vi "TDMS_Logging_Loop.vi"(6 "Logging Period (ms)":i64=20, 7 "Buffer Size":u32=1000, 9 "Group Initialization":T2(array[cluster]), 10 "TDMS Name":string="Test", 11 "Log to USB?":bool) -> ()   [LabVIEW 2015]
uses:
  <userlib>/836-Library/System/TDMSv2/Group_Data.ctl
  <userlib>/836-Library/System/TDMSv2/Group_Channels.ctl
  <userlib>/836-Library/System/TDMSv2/TDMS_RT_FIFO_Packet.ctl
  <userlib>/836-Library/System/TDMSv2/Channel_Initializer.ctl
  <vilib>/Platform/TimedLoop/XDataNode/timing_clust.ctl
  <vilib>/Platform/TimedLoop/XDataNode/nitl_modes.ctl
  <vilib>/Platform/TimedLoop/XDataNode/wakeup.ctl
  <userlib>/836-Library/System/TDMSv2/Back_Channel_Data.ctl
  <vilib>/platform/TimedLoop/XDataNode/XDataNode.xnode
  <vilib>/Platform/TimedLoop/XDataNode/XDNodeRunTimeDep.lvlib
panel:
  out "Logging Iteration Count":i32
  out "TDMS Name":string="Test"
  out "File Creation Loop Iteration":i32
  out "Current Data":T1
  out "TDMS File Location":path
  out "Cluster 2":T5
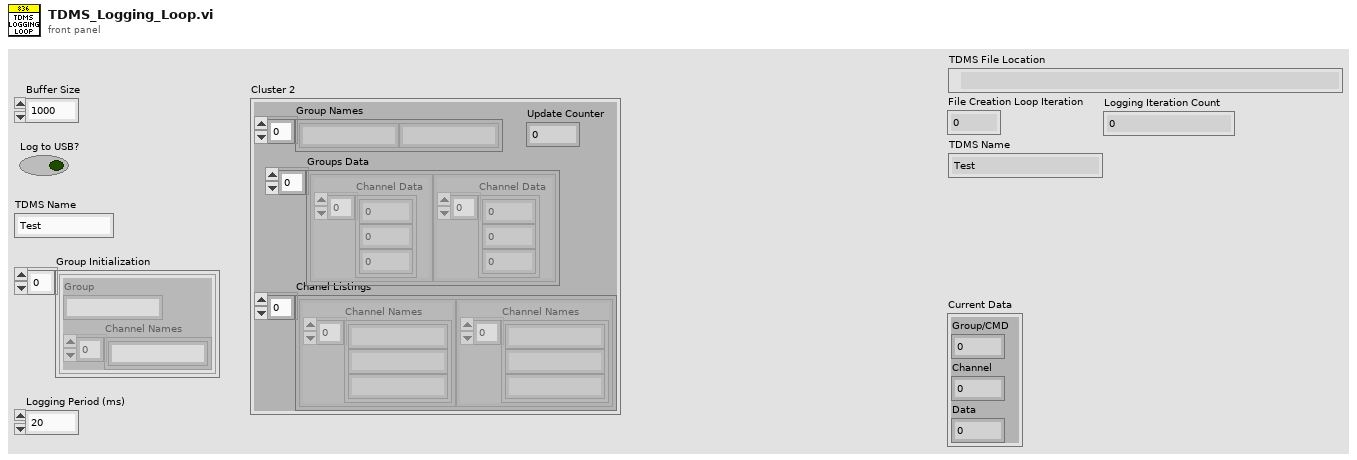
[diagram p1: front panel]
types:
  T1 = typedef "TDMS_RT_FIFO_Packet.ctl" = cluster{"Group/CMD":i32, "Channel":i32, "Data":dbl}
  T2 = cluster{"Group":string, "Channel Names":string[]}[]
  T3 = typedef "Group_Data.ctl" = cluster{"Channel Data":dbl[]}
  T4 = typedef "Group_Channels.ctl" = cluster{"Channel Names":string[]}
  T5 = cluster{"Group Names":string[], "Groups Data":T3[], "Update Counter":i32, "Chanel Listings":T4[]}
  T6 = enum16{"open", "open or create", "create or replace", "create", "open (read-only)"}
  T7 = typedef "XDNodeRunTimeDep.lvlib/timing_clust.ctl" = cluster{"Expected End [f-1]":u64, "Actual End [f-1]":u64, "Finished Late? [f-1]":bool, "Expected End [i-1]":u64, "Actual End [i-1]":u64, "Finished Late? [i-1]":bool, "Expected Start [i]":u64, "Actual Start [i]":u64, "Expected Start [f]":u64, "Actual Start [f]":u64, "Source Name":string, "Structure Name":string, "Period":i64, "Deadline":i64, "Offset":i64, "Start":i64, "Priority":i32, "Timeout":i32, "Mode":T8, "Wakeup Reason":T9, "Error":errorcluster, "Source Type":string, "Secondary Source Type":string, "Global End Time":u64, "Global Start Time":u64, "Frame Duration":u64, "Iteration Duration":u64, "Assigned CPU":i32, "I/O Scan Engine Mode":u32}
  T8 = typedef "XDNodeRunTimeDep.lvlib/nitl_modes.ctl" = enum32{"No Change", "Process missed periods, maintain original phase", "Discard missed periods, maintain original phase", "Process missed periods, ignore original phase", "Discard missed periods, ignore original phase"}
  T9 = typedef "XDNodeRunTimeDep.lvlib/wakeup.ctl" = enum32{"Normal", "Aborted", "Asynchronous wakeup", "Timing source error", "Timed loop error", "Timeout"}
  T10 = typedef "Channel_Initializer.ctl" = cluster{"Column Headers":string[], "Initialization array":dbl[]}
  T11 = typedef "Back_Channel_Data.ctl" = cluster{"Group":string, "Channel":string, "Return Notifier":refnum<notifier>}
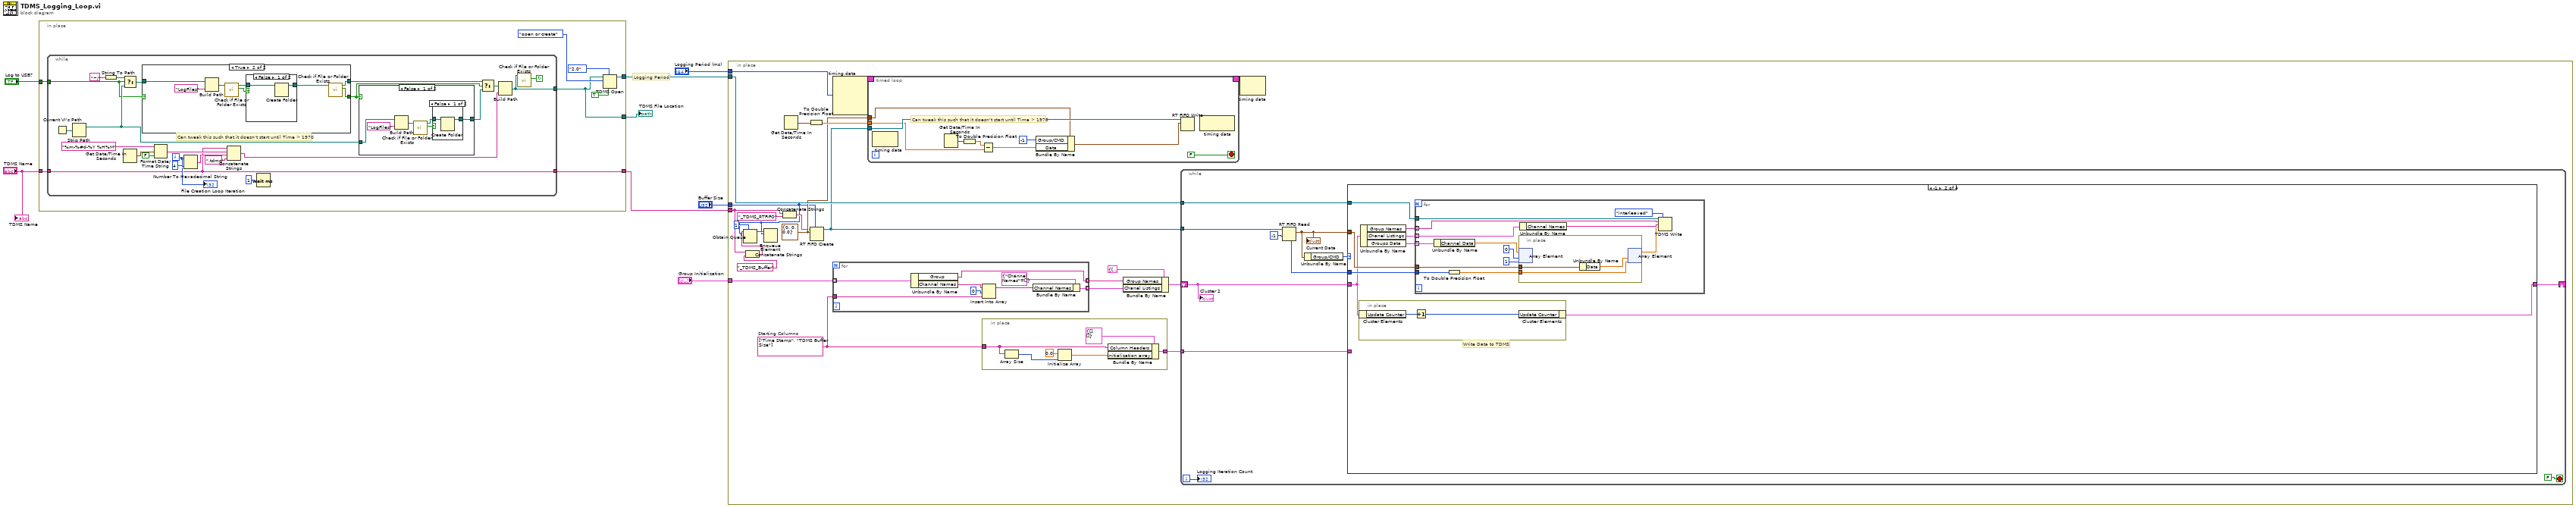
[diagram p0: block diagram]
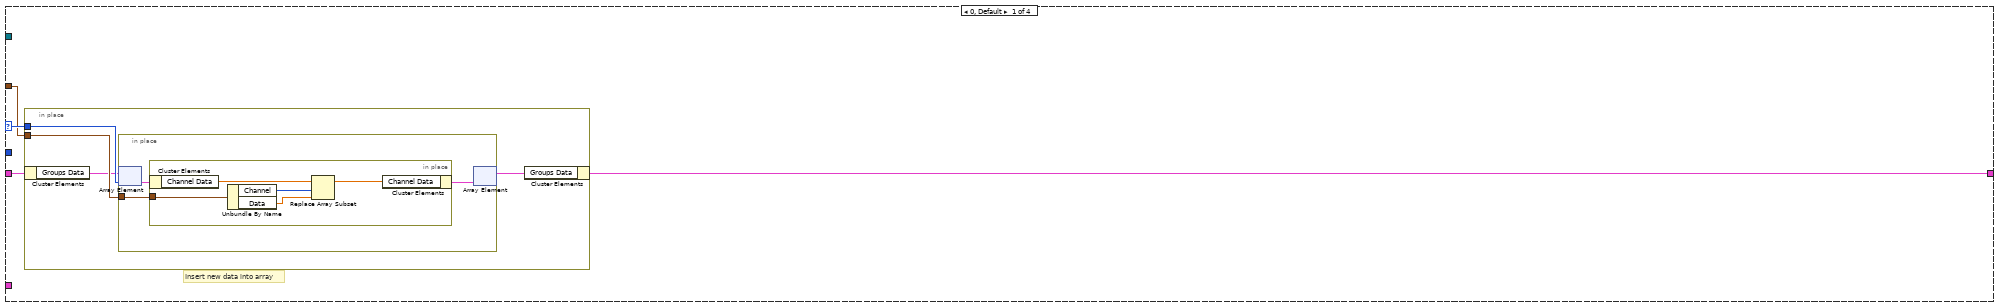
[diagram p6: hidden frame]
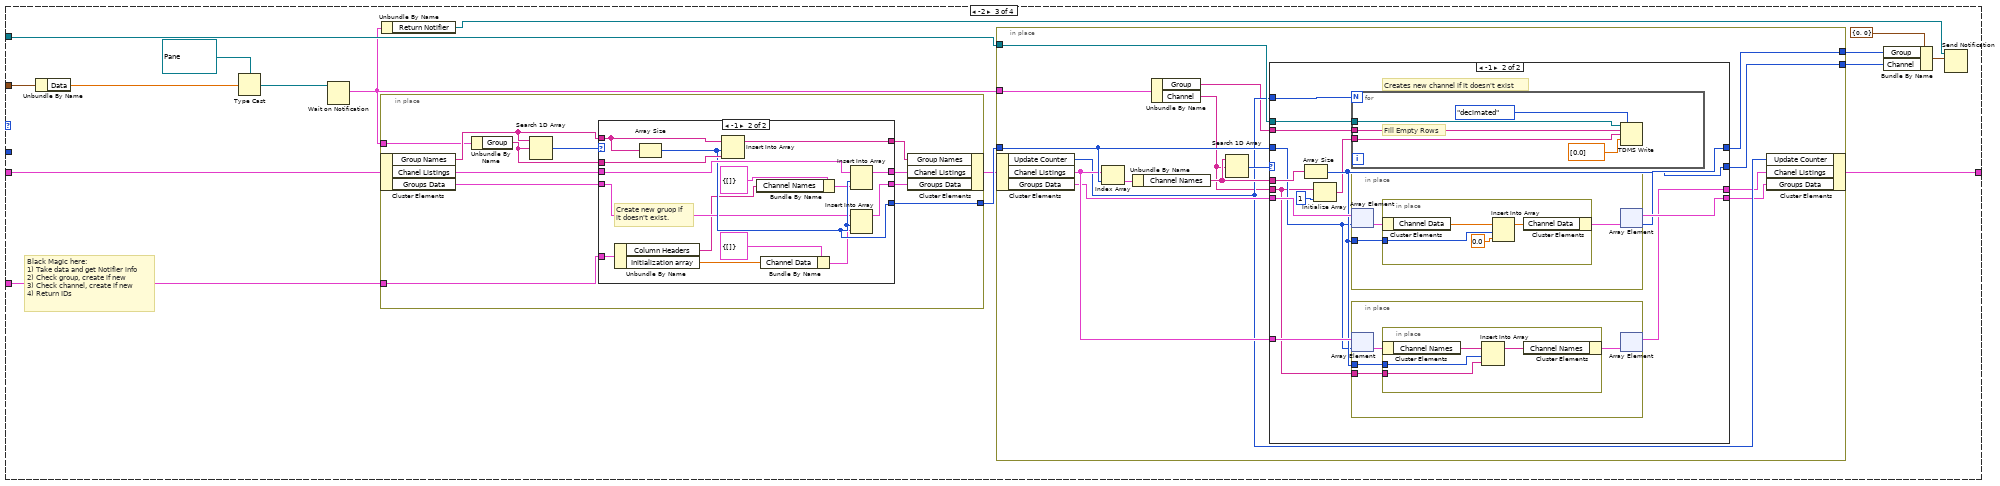
[diagram p7: hidden frame]
diagram:
  # "Logging Period"
  n1 = in-place {
    in-place-border: [w11] -> w2
    in-place-border: "Log to USB?" -> [w13]
    in-place-border: "TDMS Name" -> [w12]
    in-place-border: [w10] -> w5
    in-place-border: [w9] -> w1
    n2 = while {
      tunnel: [w29] -> w9
      tunnel: w13 -> [w18]
      tunnel: w12 -> [w17]
      tunnel: [w17] -> w10
      i -> [w33]
      stop <- w30 continue-if-true
      # "Can tweak this such that it doesn't start until Time > 1970"
      n3 = Current VI's Path() -> (path=w28:path)
      n4 = Strip Path(path=w28) -> (stripped path=w22:path)  [unwired: 1 out]
      n5 = String To Path(string="~/") -> (path=w26:path)
      n6 = Select(t=w26, s=w18, f=w22) -> (s? t:f=w27:path)
      n7 = Get Date/Time In Seconds() -> (seconds since 1Jan1904=w35:timestamp)
      n8 = case shown="True" w18 {
        selector: w18 -> [w41 _]
        tunnel: w27 -> [w40 w46]
        tunnel: [w40 w43] -> w24
        tunnel: [w41 w42] -> w21
        frame False {
        }
        frame True {
          n9 = Build Path(base path=w46, name or relative path="LogFiles") -> (appended path=w45:path)
          n10 = call <vilib>:"Check if File or Folder Exists.vi"("path"=w45) -> ("file or folder exists?"=w49:bool, "dup path"=w48:path)  [unwired: 8 in, 1 out]
          n11 = case shown="False" w49 {
            tunnel: [w51 w52] -> w44
            tunnel: w48 -> [w50 w52]
            frame False {
              n12 = Create Folder(path (use dialog)=w50) -> (created path=w51:path)  [unwired: 2 in, 2 out]
            }
            frame True {
            }
          }
          n13 = call <vilib>:"Check if File or Folder Exists.vi"("path"=w44) -> ("file or folder exists?"=w42:bool, "dup path"=w43:path)  [unwired: 8 in, 1 out]
        }
      }
      n14 = Format Date/Time String(time format string (%c)="%m-%#d-%Y %H%M", seconds (now)=w35, UTC format=FALSE) -> (date/time string=w38:string)
      n15 = Number To Hexadecimal String(1:i16 4 ("width (-)"), 2:w33) -> (0:w31:string)
      n16 = Concatenate Strings(w17, w38, w31, ".tdms" ("string")) -> (w39:string)
      n17 = Wait (ms)(milliseconds to wait=u32 1 ("millisecond multiple")) -> ()  [unwired: 1 out]
      n18 = case shown="False" w21 {
        tunnel: w22 -> [w57 w62]
        tunnel: [w53 w62] -> w20
        frame False {
          n19 = Build Path(base path=w57, name or relative path="LogFiles") -> (appended path=w54:path)
          n20 = call <vilib>:"Check if File or Folder Exists.vi"("path"=w54) -> ("file or folder exists?"=w55:bool, "dup path"=w56:path)  [unwired: 8 in, 1 out]
          n21 = case shown="False" w55 {
            tunnel: [w60 w61] -> w53
            tunnel: w56 -> [w59 w61]
            frame False {
              n22 = Create Folder(path (use dialog)=w59) -> (created path=w60:path)  [unwired: 2 in, 2 out]
            }
            frame True {
            }
          }
        }
        frame True {
        }
      }
      n23 = Select(t=w24, s=w21, f=w20) -> (s? t:f=w23:path)
      n24 = Build Path(base path=w23, name or relative path=w39) -> (appended path=w29:path)
      n25 = call <vilib>:"Check if File or Folder Exists.vi"("path"=w29) -> ("file or folder exists?"=w30:bool)  [unwired: 8 in, 2 out]
      "File Creation Loop Iteration" <- w33
    }
    n26 = TDMS Open(6:TRUE ("disable buffering? (T)"), 7:enum16{"1.0", "2.0"}."2.0" ("file format version (2.0)"), 10:T6."open or create" ("operation (0:open)"), 11:w9) -> (3:w11:refnum<k34>)  [unwired: 3 in, 1 out]
  }
  "TDMS File Location" <- w1
  n27 = in-place {
    in-place-border: w2 -> [w85]
    in-place-border: "Logging Period (ms)" -> [w81]
    in-place-border: w5 -> [w68]
    in-place-border: "Buffer Size" -> [w63]
    in-place-border: "Group Initialization" -> [w78]
    w73 = string[] ["Time Stamp", "TDMS Buffer Size"]  # Starting Columns
    w80 = T1 {"Group/CMD"=0, "Channel"=0, "Data"=0.0}
    n28 = Concatenate Strings(w68, "_TDMS_Buffer" ("string")) -> (w67:string)
    n29 = Obtain Queue(max queue size (-1, unlimited)=1, name (unnamed)=w67, element data type=w63) -> (queue out=w64:refnum<queue>)  [unwired: 2 in, 2 out]
    n30 = Enqueue Element(queue=w64, element=w63) -> ()  [unwired: 2 in, 3 out]
    n31 = Concatenate Strings(w68, "_TDMS_RTFIFO" ("string")) -> (w72:string)
    n32 = Get Date/Time In Seconds() -> (seconds since 1Jan1904=w82:timestamp)
    n33 = To Double Precision Float(number=w82) -> (double precision float=w83:dbl)
    n34 = RT FIFO Create(0:w72, 1:w80, 4:w63) -> (8:w84:refnum<k33>)  [unwired: 5 in, 2 out]
    n35 = node-c288(w81) -> (w70:T7)  [unwired: 3 in]
    n36 = for {
      tunnel: w78 -> [w108] mode=indexing
      tunnel: [w107] -> w76 mode=indexing
      tunnel: [w104] -> w74 mode=indexing
      tunnel: w73 -> [w101]
      n37 = Unbundle By Name(w108) -> ("Group"=w107:string, "Channel Names"=w106:string[])
      n38 = Insert Into Array(array=w106, index=0, new element=w101) -> (w103:string[])
      n39 = Bundle By Name(cluster=T4 {"Channel Names"=[]}, "Channel Names"=w103) -> (w104:T4)
    }
    n40 = timed-loop {
      timing: w70 -> [_]
      timing-out: [_] -> w69
      tunnel: w84 -> [w93]
      tunnel: w80 -> [w92]
      tunnel: w83 -> [w86]
      stop <- FALSE stop-if-true
      # "Can tweak this such that it doesn't start until Time > 1970"
      n41 = node-c288() -> ()  [unwired: 1 in, 1 out]
      n42 = Get Date/Time In Seconds() -> (seconds since 1Jan1904=w89:timestamp)
      n43 = To Double Precision Float(number=w89) -> (double precision float=w88:dbl)
      n44 = Subtract(x=w88, y=w86) -> (x-y=w87:dbl)
      n45 = Bundle By Name(cluster=w92, "Group/CMD"=-1 ("Index/CMD"), "Data"=w87) -> (w91:T1)
      n46 = RT FIFO Write(0:w93, 1:w91) -> ()  [unwired: 3 in, 4 out]
      n47 = node-c288() -> ()  [unwired: 1 in, 1 out]
    }
    n48 = in-place {
      in-place-border: w73 -> [w110]
      in-place-border: [w109] -> w79
      n49 = Array Size(array=w110) -> (size(s)=w113:i32)
      n50 = Initialize Array(0.0 ("element"), w113) -> (w111:dbl[])
      n51 = Bundle By Name(cluster=T10 {"Column Headers"=[], "Initialization array"=[]} ("Column Initializer"), "Column Headers"=w110, "Initialization array"=w111) -> (w109:T10)
    }
    n52 = Bundle By Name(cluster=T5 {"Group Names"=[], "Groups Data"=[], "Update Counter"=0, "Chanel Listings"=[]}, "Group Names"=w76, "Chanel Listings"=w74) -> (w75:T5)
    n53 = while {
      tunnel: w85 -> [w125]
      tunnel: w84 -> [w123]
      tunnel: w79 -> [w119]
      shift-right: [w116] -> _
      shift-left: w75 -> [w117]
      i -> [w115]
      stop <- FALSE stop-if-true
      n54 = RT FIFO Read(0:w123, 2:-1 ("timeout in ms (0)")) -> (7:w121:u32, 9:w118:T1)  [unwired: 2 in, 3 out]
      "Current Data" <- w118
      n55 = Unbundle By Name(w118) -> ("Group/CMD"=w122:i32)
      n56 = case shown="-1" w122 {
        selector: w122 -> [w129 _ _ _]
        tunnel: w125 -> [_ w149 w176 _]
        tunnel: w121 -> [_ w148 _ _]
        tunnel: w119 -> [_ _ w175 _]
        tunnel: w118 -> [w128 w147 w174 _]
        tunnel: w117 -> [w127 w143 w172 w267]
        tunnel: [w126 w142 w170 w267] -> w116
        frame 0, Default {
          # "Insert new data into array"
          n57 = in-place {
            in-place-border: w129 -> [w133]
            in-place-border: w128 -> [w132]
            n58 = in-place-cluster #1(w127) -> ("Groups Data"=w131:T3[])
            n59 = in-place {
              in-place-border: w132 -> [w134]
              n60 = in-place-array #2(w131, w133) -> (w136:T3)
              n61 = in-place {
                in-place-border: w134 -> [w139]
                n62 = in-place-cluster #3(w136) -> ("Channel Data"=w141:dbl[])
                n63 = Unbundle By Name(w139) -> ("Channel"=w138:i32, "Data"=w137:dbl)
                n64 = Replace Array Subset(array=w141, new element=w137, index=w138) -> (w140:dbl[])
                n65 = in-place-cluster #3("Channel Data"=w140) -> (w135:T3)
              }
              n66 = in-place-array #2(w135) -> (w130:T3[])  [unwired: 1 out]
            }
            n67 = in-place-cluster #1("Groups Data"=w130) -> (w126:T5)
          }
        }
        frame -1 {
          # "Write Data to TDMS"
          n68 = in-place {
            n69 = in-place-cluster #4(w143) -> ("Update Counter"=w151:i32)
            n70 = Increment(x=w151) -> (x+1=w150:i32)
            n71 = in-place-cluster #4("Update Counter"=w150) -> (w142:T5)
          }
          n72 = Unbundle By Name(w143) -> ("Group Names"=w144:string[], "Chanel Listings"=w146:T4[], "Groups Data"=w145:T3[])
          n73 = for {
            tunnel: w149 -> [w164]
            tunnel: w145 -> [w163] mode=indexing
            tunnel: w146 -> [w162] mode=indexing
            tunnel: w144 -> [w161] mode=indexing
            tunnel: w148 -> [w160]
            tunnel: w147 -> [w152]
            n74 = Unbundle By Name(w163) -> ("Channel Data"=w157:dbl[])
            n75 = To Double Precision Float(number=w160) -> (double precision float=w154:dbl)
            n76 = in-place {
              in-place-border: w154 -> [w167]
              in-place-border: w152 -> [w166]
              n77 = in-place-array #5(w157, 0, 1) -> ()  [unwired: 2 out]
              n78 = Unbundle By Name(w166) -> ("Data"=w165:dbl)
              n79 = in-place-array #5(w165, w167) -> (w153:dbl[])  [unwired: 2 out]
            }
            n80 = Unbundle By Name(w162) -> ("Channel Names"=w159:string[])
            n81 = TDMS Write(0:w164, 1:enum16{"decimated", "interleaved"}."interleaved" ("data layout (0:decimated)"), 5:w161, 7:w159, 9:w153) -> ()  [unwired: 1 in, 4 out]
          }
        }
        frame -2 {
          # "Black Magic here:\n1) Take data and get Notifier info\n2) Check group, create if new\n3) Check channel, create if new\n4) Return IDs"
          n82 = Unbundle By Name(w174) -> ("Data"=w173:dbl)
          n83 = Type Cast(type=refnum<notifier> refnum ("notifier out"), x=w173) -> (*(type *) &x=w182:refnum<notifier>)
          n84 = Wait on Notification(notifier=w182) -> (notification=w168:T11)  [unwired: 3 in, 3 out]
          n85 = in-place {
            in-place-border: [w246] -> w178
            in-place-border: w175 -> [w245]
            in-place-border: w168 -> [w238]
            n86 = in-place-cluster #6(w172) -> ("Group Names"=w244:string[], "Chanel Listings"=w240:T4[], "Groups Data"=w242:T3[])
            n87 = Unbundle By Name(w238) -> ("Group"=w237:string)
            n88 = Search 1D Array(1D array=w244, element=w237) -> (index of element=w247:i32)  [unwired: 1 in]
            n89 = case shown="-1" w247 {
              selector: w247 -> [w251 _]
              tunnel: w244 -> [w250 w266]
              tunnel: w237 -> [_ w265]
              tunnel: [w251 w262] -> w246
              tunnel: [w250 w264] -> w243
              tunnel: w240 -> [w249 w263]
              tunnel: w242 -> [w248 w261]
              tunnel: [w249 w260] -> w239
              tunnel: [w248 w259] -> w241
              tunnel: w245 -> [_ w254]
              frame 0, Default {
              }
              frame -1 {
                # "Create new gruop if\nit doesn't exist."
                n90 = Unbundle By Name(w254) -> ("Column Headers"=w252:string[], "Initialization array"=w253:dbl[])
                n91 = Array Size(array=w266) -> (size(s)=w262:i32)
                n92 = Insert Into Array(array=w266, index=w262, new element=w265) -> (w264:string[])
                n93 = Bundle By Name(cluster=T4 {"Channel Names"=[]}, "Channel Names"=w252) -> (w255:T4)
                n94 = Bundle By Name(cluster=T3 {"Channel Data"=[]} ("new element/subarray"), "Channel Data"=w253) -> (w257:T3)
                n95 = Insert Into Array(array=w263, index=w262, new element=w255) -> (w260:T4[])
                n96 = Insert Into Array(array=w261, index=w262, new element=w257) -> (w259:T3[])
              }
            }
            n97 = in-place-cluster #6("Group Names"=w243, "Chanel Listings"=w239, "Groups Data"=w241) -> (w171:T5)
          }
          n98 = Unbundle By Name(w168) -> ("Return Notifier"=w169:refnum<notifier>)
          n99 = in-place {
            in-place-border: [w197] -> w179
            in-place-border: w178 -> [w194]
            in-place-border: [w193] -> w177
            in-place-border: w176 -> [w192]
            in-place-border: w168 -> [w186]
            n100 = in-place-cluster #7(w171) -> ("Update Counter"=w189:i32, "Chanel Listings"=w191:T4[], "Groups Data"=w190:T3[])
            n101 = Index Array(array=w191, index=w194) -> (element=w196:T4)
            n102 = Unbundle By Name(w196) -> ("Channel Names"=w195:string[])
            n103 = Unbundle By Name(w186) -> ("Group"=w184:string, "Channel"=w185:string)
            n104 = Search 1D Array(1D array=w195, element=w185) -> (index of element=w198:i32)  [unwired: 1 in]
            n105 = case shown="-1" w198 {
              selector: w198 -> [w201 _]
              tunnel: [w202 w210] -> w188
              tunnel: w191 -> [w202 w212]
              tunnel: [w201 w211] -> w197
              tunnel: [w200 w214] -> w187
              tunnel: w190 -> [w200 w215]
              tunnel: w195 -> [_ w216]
              tunnel: w194 -> [w199 w209]
              tunnel: [w199 w213] -> w193
              tunnel: w185 -> [_ w205]
              tunnel: w189 -> [_ w208]
              tunnel: w184 -> [_ w207]
              tunnel: w192 -> [_ w203]
              frame 0, Default {
              }
              frame -1 {
                # "Creates new channel if it doesn't exist"
                n106 = Array Size(array=w216) -> (size(s)=w211:i32)
                n107 = Initialize Array(w205, 1 ("dimension size")) -> (w204:string[])
                n108 = for {
                  N: w208 -> [_]
                  tunnel: w207 -> [w220]
                  tunnel: w204 -> [w219]
                  tunnel: w203 -> [w217]
                  # "Fill Empty Rows"
                  n109 = TDMS Write(0:w217, 1:enum16{"decimated", "interleaved"}."decimated" ("data layout (0:decimated)"), 5:w220, 7:w219, 9:dbl[] [0.0]) -> ()  [unwired: 1 in, 4 out]
                }
                n110 = in-place {
                  in-place-border: w211 -> [w230]
                  n111 = in-place-array #8(w215, w209) -> (w232:T3)
                  n112 = in-place {
                    in-place-border: w230 -> [w235]
                    n113 = in-place-cluster #9(w232) -> ("Channel Data"=w236:dbl[])
                    n114 = Insert Into Array(array=w236, index=w235, new element=0.0 ("new element/subarray")) -> (w233:dbl[])
                    n115 = in-place-cluster #9("Channel Data"=w233) -> (w231:T3)
                  }
                  n116 = in-place-array #8(w231) -> (w214:T3[], w213:i32)
                }
                n117 = in-place {
                  in-place-border: w211 -> [w223]
                  in-place-border: w205 -> [w222]
                  n118 = in-place-array #10(w212, w209) -> (w225:T4)
                  n119 = in-place {
                    in-place-border: w223 -> [w228]
                    in-place-border: w222 -> [w226]
                    n120 = in-place-cluster #11(w225) -> ("Channel Names"=w229:string[])
                    n121 = Insert Into Array(array=w229, index=w228, new element=w226) -> (w227:string[])
                    n122 = in-place-cluster #11("Channel Names"=w227) -> (w224:T4)
                  }
                  n123 = in-place-array #10(w224) -> (w210:T4[])  [unwired: 1 out]
                }
              }
            }
            n124 = in-place-cluster #7("Update Counter"=w189, "Chanel Listings"=w188, "Groups Data"=w187) -> (w170:T5)
          }
          n125 = Bundle By Name(cluster=cluster{"Group":i32, "Channel":i32} {"Group"=0, "Channel"=0} ("notification"), "Group"=w177, "Channel"=w179) -> (w180:cluster{"Group":i32, "Channel":i32})
          n126 = Send Notification(notification=w180, notifier=w169) -> ()  [unwired: 1 in, 2 out]
        }
        frame -3 {
          # "Do Nothing"
        }
      }
      "Cluster 2" <- w117
      "Logging Iteration Count" <- w115
    }
    n127 = node-c288(w69) -> ()  [unwired: 1 out]
  }
  "TDMS Name" <- "TDMS Name"
